vi "Start Sequential Monitor if Not Started.vi"(8 "error in":errorcluster, 11 "core handle in":u64) -> (0 "error out":errorcluster, 3 "core handle out":u64)   [LabVIEW 2020, in "AIM ARINC 429 Engine.lvlib" / "Custom Device.lvlib"]
uses:
  Custom Device.lvlib
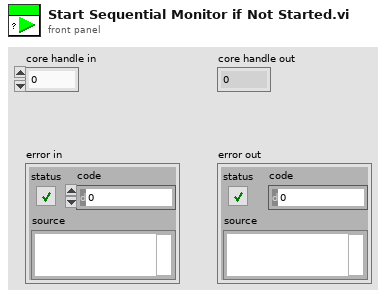
[diagram p1: front panel]
types:
  T1 = typedef "BTICardLV.lvlib/Seq Run Status.ctl" = u32
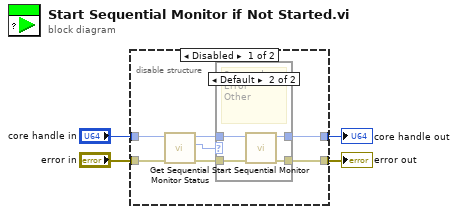
[diagram p0: block diagram]
diagram:
  n1 = disable-structure shown="Disabled" {
    disable-tunnel: "core handle in" -> [w10 w19]
    disable-tunnel: "error in" -> [w7 w18]
    disable-tunnel: [w6 w18] -> w2
    disable-tunnel: [w5 w19] -> w1
    frame Disabled {
      n2 = call <instrlib>:"Get Sequential Monitor Status.vi"("error in (no error)"=w7, "core handle in"=w10) -> ("error out"=w8:errorcluster, "run status"=w9:T1, "core handle out"=w11:u64)  [unwired: 6 in, 1 out]
      n3 = case shown="Default" w9 {
        tunnel: w8 -> [w13 w17]
        tunnel: [w13 w16] -> w6
        tunnel: w11 -> [w12 w15]
        tunnel: [w12 w14] -> w5
        frame 0 {
          # "Started"
        }
        frame Default {
          # "Stopped\nError\nOther"
          n4 = call <instrlib>:"Start Sequential Monitor.vi"("error in (no error)"=w17, "core handle in"=w15) -> ("error out"=w16:errorcluster, "core handle out"=w14:u64)  [unwired: 8 in]
        }
      }
    }
    frame Enabled {
    }
  }
  "error out" <- w2
  "core handle out" <- w1
